vi "SVM_GridSearch_FromFile.vi"() -> ()   [LabVIEW 2014]
uses:
  Controls/Options Training.ctl
  Controls/Parameters C_SVC.ctl
  Tools/Controls/Binary_ConfusionMatrix.ctl
  Controls/Kernel.ctl
  Wrapper API/Controls/svm_kernel_type.ctl
  SubVIs/SVM Train C_SVC.vi
  Tools/SubVIs/Sparse - Scale Nodes Linear.vi
  Tools/SubVIs/Sparse - Scale Problem Linear.vi
  Wrapper API/svm_train.vi
  Wrapper API/svm_predict.vi
panel:
  out "Gridsearch time (ms)":u32
  out "log2(gamma) max":dbl
  out "log2(C) max":dbl
  out "error out":errorcluster
  out "Binary Confusion Matrix":T1
  out "Misclassification counts":i32[](array[numeric])
  in  "libsvm":T4={"libsvm options"={"cache_size"=200.0, "eps"=0.001, "shrinking"=TRUE, "probability"=FALSE}, "libsvm weights"={"C"=1.0, "weight_label"=[], "weight"=[]}}
  in  "Grid parameters":T5={"C start"=-5.0, "C end"=15.0, "C step"=4.0, "Gamma start"=-15.0, "Gamma end"=3.0, "Gamma step"=4.0, "K"=10, "random seed"=-1}
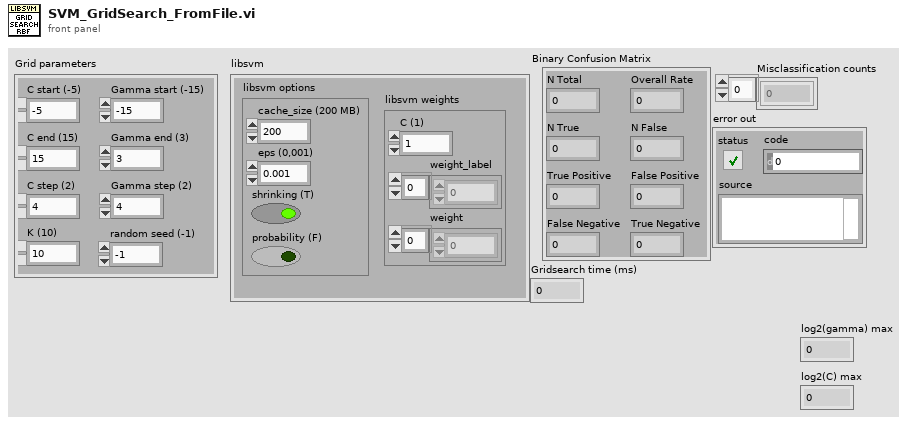
[diagram p1: front panel]
types:
  T1 = typedef "Binary_ConfusionMatrix.ctl" = cluster{"N Total":u32, "N True":u32, "N False":u32, "Overall Rate":dbl, "True Positive":dbl, "False Positive":dbl, "False Negative":dbl, "True Negative":dbl}
  T2 = typedef "Options Training.ctl" = cluster{"cache_size":dbl, "eps":dbl, "shrinking":bool, "probability":bool}
  T3 = typedef "Parameters C_SVC.ctl" = cluster{"C":dbl, "weight_label":i32[], "weight":dbl[]}
  T4 = cluster{"libsvm options":T2, "libsvm weights":T3}
  T5 = cluster{"C start":dbl, "C end":dbl, "C step":dbl, "Gamma start":dbl, "Gamma end":dbl, "Gamma step":dbl, "K":i32, "random seed":i32}
  T6 = typedef "svm_kernel_type.ctl" = enum32{"LINEAR", "POLY", "RBF", "SIGMOID", "PRECOMPUTED"}
  T7 = typedef "Kernel.ctl" = cluster{"Type":T6, "Degree":i32, "Gamma":dbl, "Coef0":dbl}
  T8 = typedef "svm_problem.ctl" = cluster{"y":dbl[], "x":cluster{T9[]}[]}
  T9 = typedef "svm_node.ctl" = cluster{"index":i32, "value":dbl}
  T10 = typedef "svm_model.ctl" = cluster{"param":T11, "nr_class":i32, "l":i32, "SV":cluster{"Array":T9[]}[], "sv_coef":dbl[][], "rho":dbl[], "probA":dbl[], "probB":dbl[], "sv_indices":i32[], "label":i32[], "nSV":i32[]}
  T11 = typedef "svm_parameter.ctl" = cluster{"svm_type":T12, "kernel_type":T6, "degree":i32, "gamma":dbl, "coef0":dbl, "cache_size":dbl, "eps":dbl, "C":dbl, "weight_label":i32[], "weight":dbl[], "nu":dbl, "p":dbl, "shrinking":bool, "probability":bool}
  T12 = typedef "svm_type.ctl" = enum32{"C_SVC", "NU_SVC", "ONE_CLASS", "EPSILON_SVR", "NU_SVR"}
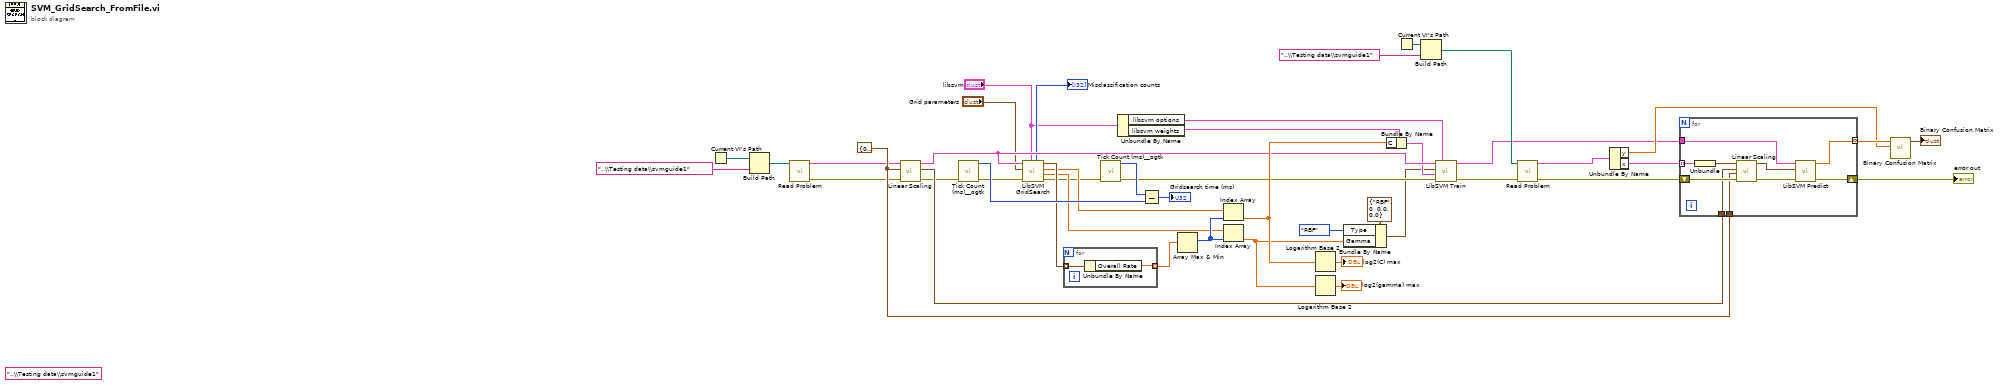
[diagram p0: block diagram]
diagram:
  (unwired) "..\\Testing data\\svmguide1"
  w35 = cluster{"X lower":dbl, "X upper":dbl} {"X lower"=0.0, "X upper"=1.0} ("X Scaling limits")
  n1 = Current VI's Path() -> (path=w45:path)
  n2 = Build Path(base path=w45, name or relative path="..\\Testing data\\svmguide1") -> (appended path=w26:path)
  n3 = call "Read Problem.vi"("file path (use dialog)"=w26) -> ("error out"=w20:errorcluster, "svm_problem"=w21:T8)  [unwired: 9 in]
  n4 = call-poly "Linear Scaling.vi"("error in (no error)"=w20, "X Scaling limits"=w35, "Problem"=w21) -> ("error out"=w25:errorcluster, "xmaxmin"=w36:cluster{"min":dbl, "max":dbl}[], "Scaled problem"=w17:T8)  [unwired: 5 in, 1 out]
  n5 = call <userlib>:"Tick Count (ms)__ogtk.vi"("error in (no error)"=w25) -> ("error out"=w16:errorcluster, "millisecond timer value"=w23:u32)  [unwired: 9 in]
  n6 = call "LibSVM GridSearch.vi"("libsvm"="libsvm", "error in (no error)"=w16, "Grid parameters"="Grid parameters", "Problem"=w17) -> ("error out"=w11:errorcluster, "gamma"=w12:dbl[], "C"=w13:dbl[], "Confusion matrices"=w14:T1[], "Misclassification counts"=→"Misclassification counts":i32[])  [unwired: 3 in]
  n7 = for {
    tunnel: w14 -> [w47] mode=indexing
    tunnel: [w46] -> w44 mode=indexing
    n8 = Unbundle By Name(w47) -> ("Overall Rate"=w46:dbl)
  }
  n9 = call <userlib>:"Tick Count (ms)__ogtk.vi"("error in (no error)"=w11) -> ("error out"=w8:errorcluster, "millisecond timer value"=w24:u32)  [unwired: 9 in]
  n10 = Unbundle By Name("libsvm") -> ("libsvm options"=w5:T2, "libsvm weights"=w42:T3)
  n11 = Subtract(x=w24, y=w23) -> (x-y=→"Gridsearch time (ms)":u32)
  n12 = Array Max & Min(array=w44) -> (max index (indices)=w43:i32)  [unwired: 3 out]
  n13 = Index Array(array=w13, index=w43) -> (element=w30:dbl)
  n14 = Index Array(array=w12, index=w43) -> (element=w29:dbl)
  n15 = Logarithm Base 2(1:w29) -> (0:→"log2(gamma) max":dbl)
  n16 = Logarithm Base 2(1:w30) -> (0:→"log2(C) max":dbl)
  n17 = Bundle By Name(cluster=T7 {"Type"=enum."RBF", "Degree"=0, "Gamma"=0.0, "Coef0"=0.0} ("Kernel"), "Type"=svm_kernel_type."RBF", "Gamma"=w29) -> (w6:T7)
  n18 = Bundle By Name(cluster=w42, "C"=w30) -> (w7:T3)
  n19 = Current VI's Path() -> (path=w39:path)
  n20 = Build Path(base path=w39, name or relative path="..\\Testing data\\svmguide1") -> (appended path=w38:path)
  n21 = call-poly "LibSVM Train.vi"("Options"=w5, "error in (no error)"=w8, "Param C_SVC"=w7, "Kernel"=w6, "Problem"=w17) -> ("error out"=w3:errorcluster, "Model"=w4:T10)  [unwired: 5 in]
  n22 = call "Read Problem.vi"("error in (no error)"=w3, "file path (use dialog)"=w38) -> ("error out"=w18:errorcluster, "svm_problem"=w19:T8)  [unwired: 8 in]
  n23 = Unbundle By Name(w19) -> ("y"=w33:dbl[], "x"=w37:cluster{T9[]}[])
  n24 = for {
    tunnel: w37 -> [w57] mode=indexing
    tunnel: w36 -> [w54]
    tunnel: w35 -> [w53]
    tunnel: w4 -> [w52]
    shift-right: [w50] -> w31
    shift-left: w18 -> [w55]
    tunnel: [w49] -> w34 mode=indexing
    n25 = Unbundle(w57) -> (w56:T9[])
    n26 = call-poly "Linear Scaling.vi"("error in (no error)"=w55, "Scaling limits"=w53, "xmaxmin"=w54, "x"=w56) -> ("error out"=w51:errorcluster, "x scaled"=w48:T9[])  [unwired: 6 in]
    n27 = call-poly "LibSVM Predict.vi"("error in (no error)"=w51, "X"=w48, "Model"=w52) -> ("error out"=w50:errorcluster, "Predicted label"=w49:dbl)  [unwired: 7 in]
  }
  "error out" <- w31
  n28 = call "Binary Confusion Matrix.vi"("Actual Labels"=w33, "Predicted Labels"=w34) -> ("Binary Confusion Matrix"=→"Binary Confusion Matrix":T1)  [unwired: 9 in]
